vi "Producer Consumer.vi"() -> ()   [LabVIEW 2018]
doc: "Use this template to build a producer/consumer design pattern. Use this template when you need to execute a process, such as data analysis, when a data source, such as a triggered acquisition, produces data at an uneven rate and you need to execute the process when the data becomes available."
uses:
  Message.ctl
panel:
  in  "Do Action":bool
  in  "stop":bool
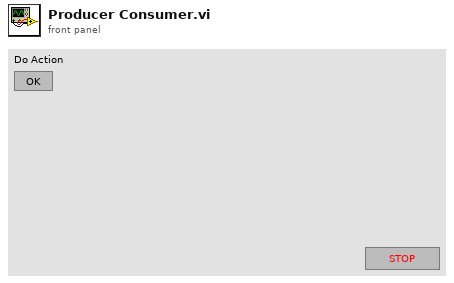
[diagram p1: front panel]
types:
  T1 = typedef "Message.ctl" = cluster{"Action":string, "Data":variant}
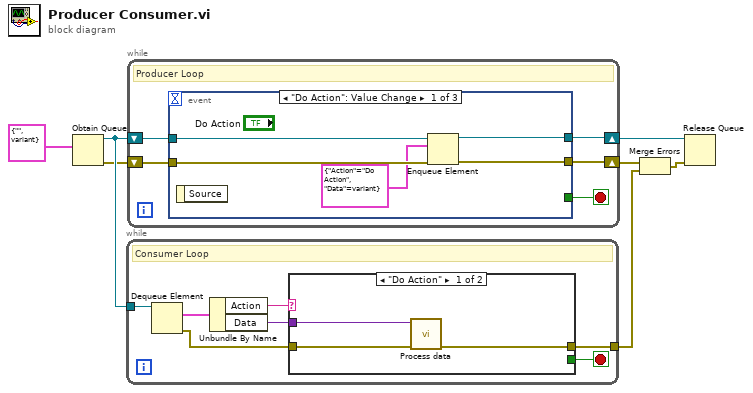
[diagram p0: block diagram]
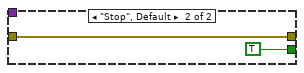
[diagram p2: hidden frame]
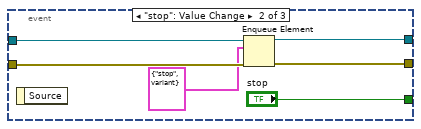
[diagram p3: hidden frame]
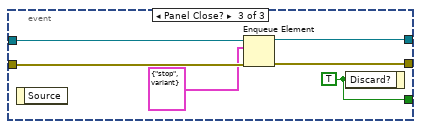
[diagram p4: hidden frame]
diagram:
  n1 = Obtain Queue(element data type=T1 {"Action"="", "Data"=variant} ("Message")) -> (queue out=w7:refnum<queue>, error out=w6:errorcluster)  [unwired: 4 in, 1 out]
  n2 = while {
    tunnel: w7 -> [w14]
    tunnel: [w8] -> w1
    stop <- w13 stop-if-true
    # "Consumer Loop"
    n3 = Dequeue Element(queue=w14) -> (element=w12:T1, error out=w9:errorcluster)  [unwired: 2 in, 2 out]
    n4 = Unbundle By Name(w12) -> ("Action"=w11:string, "Data"=w10:variant)
    n5 = case shown="\"Do Action\"" w11 {
      tunnel: [_ TRUE] -> w13
      tunnel: w10 -> [w17 _]
      tunnel: w9 -> [w16 w18]
      tunnel: [w15 w18] -> w8
      frame "Do Action" {
        n6 = call "Process data.vi"("error in (no error)"=w16, "Data"=w17) -> ("error out"=w15:errorcluster)  [unwired: 9 in]
      }
      frame "Stop", Default {
      }
    }
  }
  n7 = while {
    shift-right: [w21] -> w4
    shift-left: w6 -> [w22]
    shift-right: [w23] -> w5
    shift-left: w7 -> [w24]
    stop <- w20 stop-if-true
    # "Producer Loop"
    n8 = event shown="[0] \"Do Action\": Value Change" {
      selector: _ -> [_ _ _]
      dyn-events: _ -> [_ _ _]
      timeout: _ -> [_ _ _]
      tunnel: w24 -> [w29 w34 w41]
      tunnel: [w28 w33 w40] -> w23
      tunnel: w22 -> [w27 w31 w38]
      tunnel: [w26 w32 w39] -> w21
      tunnel: [_ "stop" w36] -> w20
      event "Do Action": Value Change {
        n9 = event-data() -> ()  [unwired: 1 in, 1 out]
        n10 = Enqueue Element(queue=w29, element=T1 {"Action"="Do Action", "Data"=variant} ("Message"), error in (no error)=w27) -> (queue out=w28:refnum<queue>, error out=w26:errorcluster)  [unwired: 1 in, 1 out]
      }
      event "stop": Value Change {
        n11 = event-data() -> ()  [unwired: 1 in, 1 out]
        n12 = Enqueue Element(queue=w34, element=T1 {"Action"="stop", "Data"=variant} ("Message"), error in (no error)=w31) -> (queue out=w33:refnum<queue>, error out=w32:errorcluster)  [unwired: 1 in, 1 out]
      }
      event Panel Close? {
        w36 = TRUE ("Discard?")
        n13 = event-data() -> ()  [unwired: 1 in, 1 out]
        n14 = Enqueue Element(queue=w41, element=T1 {"Action"="stop", "Data"=variant} ("Message"), error in (no error)=w38) -> (queue out=w40:refnum<queue>, error out=w39:errorcluster)  [unwired: 1 in, 1 out]
        n15 = event-data("Discard?"=w36) -> ()  [unwired: 1 in, 1 out]
      }
    }
  }
  n16 = Merge Errors(w4, w1) -> (w2:errorcluster)
  n17 = Release Queue(queue=w5, error in (no error)=w2) -> ()  [unwired: 1 in, 3 out]
